vi "Dispense on baseplate v2.vi"   [LabVIEW 2016]
uses:
  Classes/Routine/Dispense/Iterative Dispense/8 inch/8 inch Baseplate Dispense.lvclass
  C:/Users/HEP Gantry/Documents/GitHub/UCSB-Gantry/V5/Classes/Routine/Routine.lvclass
  Classes/Workspace/Carrier Tray/Syringe Space/Syringe Space.lvclass
  C:/Users/HEP Gantry/Documents/GitHub/UCSB-Gantry/V5/Classes/Workspace/Fixture.lvclass
  Classes/Routine/Secure Syringe/SecureRelease Syringe.lvclass
  Classes/Workspace/Pick Up Tool Area/Pick Up Tool.lvclass
  Classes/Workspace/Carrier Tray/Assembly Tray.lvclass
  Classes/Routine/Pick and Place/Pick and Place Type.ctl
  Classes/Routine/Pick and Place/Pick and Place.lvclass
  Classes/Routine/Pick and Place/Pick and Place.lvclass/Pick and Place.ctl
  Classes/Routine/Secure Syringe/SecureRelease Syringe.lvclass/SecureRelease Syringe.ctl
  Classes/Routine/Pick and Place/Write Pick and Place Type.vi
  Classes/Routine/Secure Syringe/Write Type.vi
  Classes/Workspace/Fixture.lvclass
  Classes/Routine/Routine.lvclass
  Classes/Controller/Controller.lvclass
types:
  T1 = typedef "Pick and Place.lvclass/Pick and Place Type.ctl" = enum16{"Primary Pick Up", "Secondary Pick Up", "Put Down All", "Pick Up All", "Put Down Secondary"}
  T2 = typedef "Controller.lvclass/Controllers.ctl" = cluster{"I-O.lvclass":refnum<class "I-O.lvclass">, "Motion.lvclass":refnum<class "Motion.lvclass">, "Dispenser.lvclass":refnum<class "Dispenser.lvclass">}
  T3 = typedef "Fixture.lvclass/Workspace.ctl" = cluster{"XYZTheta":dbl[], "Workspace Valve":i32, "Workspace Sensor":i32}
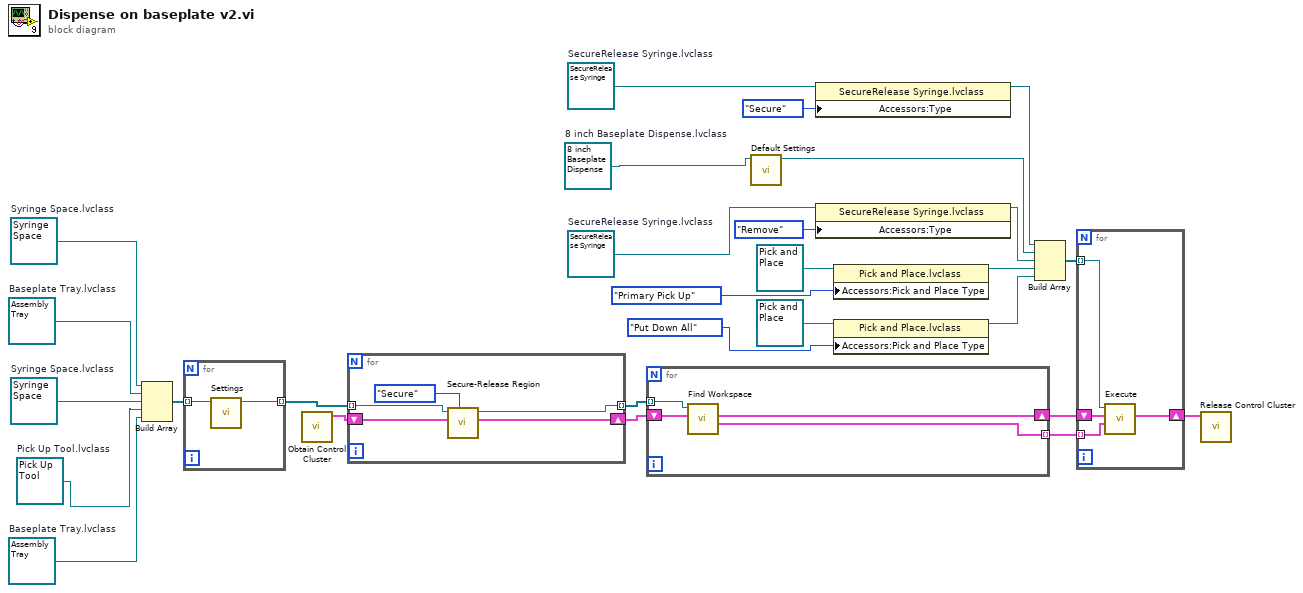
[diagram p0: block diagram]
diagram:
  w5 = refnum<class "Assembly Tray.lvclass"> refnum  # Baseplate Tray.lvclass
  w3 = refnum<class "Pick Up Tool.lvclass"> refnum  # Pick Up Tool.lvclass
  w17 = refnum<class "SecureRelease Syringe.lvclass"> refnum  # SecureRelease Syringe.lvclass
  w19 = refnum<class "SecureRelease Syringe.lvclass"> refnum  # SecureRelease Syringe.lvclass
  w26 = refnum<class "Syringe Space.lvclass"> refnum  # Syringe Space.lvclass
  w28 = refnum<class "Syringe Space.lvclass"> refnum  # Syringe Space.lvclass
  w27 = refnum<class "Assembly Tray.lvclass"> refnum  # Baseplate Tray.lvclass
  w2 = refnum<class "8 inch Baseplate Dispense.lvclass"> refnum  # 8 inch Baseplate Dispense.lvclass
  n1 = Build Array(w28, w27, w26, w3, w5) -> (w25:refnum<class "Fixture.lvclass">[])
  n2 = for {
    tunnel: w25 -> [w30] mode=indexing
    tunnel: [w29] -> w24 mode=indexing
    n3 = call-dynamic "Settings.vi"("Workspace in"=w30) -> ("Workspace out"=w29:refnum<class "Fixture.lvclass">)  [unwired: 9 in, 1 out]
  }
  n4 = call "Obtain Control Cluster.vi"() -> ("Control Out"=w22:T2)  [unwired: 11 in]
  n5 = for {
    tunnel: w24 -> [w35] mode=indexing
    tunnel: [w34] -> w23 mode=indexing
    shift-right: [w32] -> w21
    shift-left: w22 -> [w33]
    n6 = call-dynamic "Secure-Release Region.vi"("Action"=enum16{"Secure", "Release"}."Secure", "Control In"=w33, "Fixture in"=w35) -> ("Control Out"=w32:T2, "Fixture out"=w34:refnum<class "Fixture.lvclass">)  [unwired: 6 in, 1 out]
  }
  n7 = for {
    tunnel: w23 -> [w39] mode=indexing
    shift-right: [w37] -> w20
    shift-left: w21 -> [w38]
    tunnel: [w36] -> w11 mode=indexing
    n8 = call-dynamic "Find Workspace.vi"("Control In"=w38, "Workspace In"=w39) -> ("Workspace Out"=w36:T3, "Control Out"=w37:T2)  [unwired: 6 in, 2 out]
  }
  n9 = call-dynamic "Default Settings.vi"("C4 Dispense in 2"=w2) -> ("C4 Dispense out 2"=w1:refnum<class "8 inch Baseplate Dispense.lvclass">)  [unwired: 9 in, 1 out]
  n10 = property class="SecureRelease Syringe.lvclass"(reference=w19, "Accessors:Type"=enum16{"Secure", "Remove"}."Secure" ("Type")) -> (reference out=w15:refnum<class "SecureRelease Syringe.lvclass">)  [unwired: 1 in, 1 out]
  n11 = property class="SecureRelease Syringe.lvclass"(reference=w17, "Accessors:Type"=enum16{"Secure", "Remove"}."Remove" ("Type")) -> (reference out=w14:refnum<class "SecureRelease Syringe.lvclass">)  [unwired: 1 in, 1 out]
  n12 = property class="Pick and Place.lvclass"(reference=refnum<class "Pick and Place.lvclass"> refnum ("Pick and Place.lvclass"), "Accessors:Pick and Place Type"=Pick_and_Place_Type."Primary Pick Up" ("Pick and Place Type")) -> (reference out=w6:refnum<class "Pick and Place.lvclass">)  [unwired: 1 in, 1 out]
  n13 = property class="Pick and Place.lvclass"(reference=refnum<class "Pick and Place.lvclass"> refnum ("Pick and Place.lvclass"), "Accessors:Pick and Place Type"=Pick_and_Place_Type."Put Down All" ("Pick and Place Type")) -> (reference out=w4:refnum<class "Pick and Place.lvclass">)  [unwired: 1 in, 1 out]
  n14 = Build Array(w15, w1, w14, w6, w4) -> (w13:refnum<class "Routine.lvclass">[])
  n15 = for {
    tunnel: w13 -> [w42] mode=indexing
    shift-right: [w41] -> w12
    shift-left: w20 -> [w43]
    tunnel: w11 -> [w40] mode=indexing
    n16 = call-dynamic "Execute.vi"("Workspace"=w40, "Control In"=w43, "Routine in"=w42) -> ("Control Out"=w41:T2)  [unwired: 6 in, 2 out]
  }
  n17 = call "Release Control Cluster.vi"("output cluster"=w12) -> ()  [unwired: 11 in]
